vi "Export Graph.vi"(11 "Abstract Graph in":refnum<class "Abstract Graph.lvclass">) -> (3 "Abstract Graph out":refnum<class "Abstract Graph.lvclass">)   [LabVIEW 2021, in "GraphLib.lvlib" / "Abstract Graph.lvclass"]
uses:
  Abstract Graph.lvclass
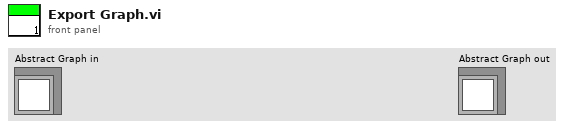
[diagram p1: front panel]
types:
  T1 = typedef "GraphLib.lvlib/Node Internal.ctl" = cluster{"Node":T2, "Edge IDs":set{string}}
  T2 = typedef "GraphLib.lvlib/Node.ctl" = cluster{"Value":variant, "Attributes":map{string, variant}}
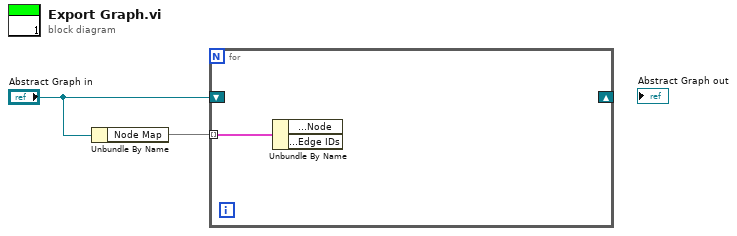
[diagram p0: block diagram]
diagram:
  n1 = Unbundle By Name("Abstract Graph in") -> ("Node Map"=w2:map{string, T1})
  n2 = for {
    tunnel: w2 -> [w3] mode=indexing
    shift-right: _ -> [_]
    shift-left: "Abstract Graph in" -> [_]
    n3 = Unbundle By Name(w3) -> ()  [unwired: 2 out]
  }
